vi "TCPcom.vi"(5 "string":string, 11 "error in":errorcluster, 13 "task":T1) -> (6 "data out":string, 15 "error out":errorcluster)   [LabVIEW 2020]
uses:
  task.ctl
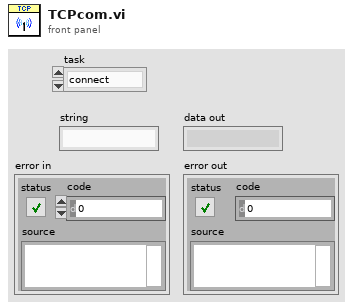
[diagram p1: front panel]
types:
  T1 = typedef "task.ctl" = enum16{"connect", "send", "send-recv", "receive", "disconnect"}
  T2 = enum16{"Standard", "Buffered", "CRLF", "Immediate"}
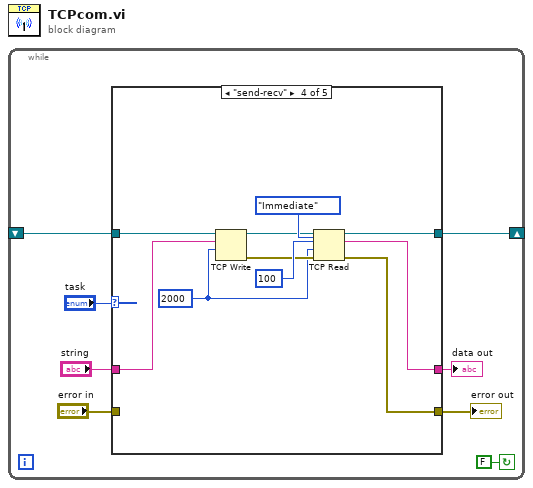
[diagram p0: block diagram]
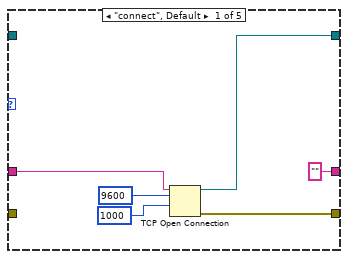
[diagram p2: hidden frame]
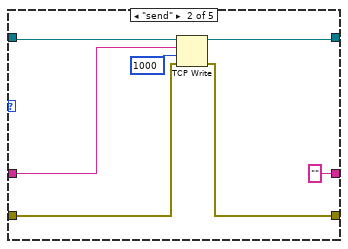
[diagram p3: hidden frame]
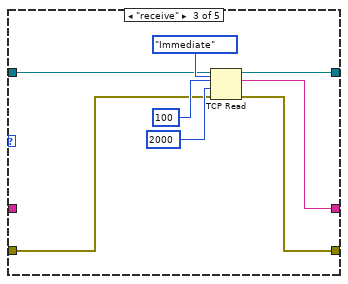
[diagram p4: hidden frame]
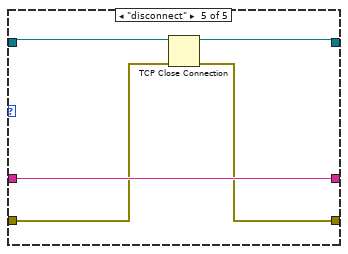
[diagram p5: hidden frame]
diagram:
  n1 = while {
    shift-right: [w7] -> _
    shift-left: _ -> [w6]
    stop <- FALSE continue-if-true
    n2 = case shown="\"send-recv\"" "task" {
      tunnel: [w10 w19 w27 w37 w42] -> w7
      tunnel: w6 -> [_ w20 w22 w34 w43]
      tunnel: "string" -> [w12 w16 _ w30 w44]
      tunnel: [w11 w17 w26 w36 w40] -> w3
      tunnel: ["" ("string") "" ("string") w25 w35 w44] -> w2
      tunnel: "error in" -> [_ w18 w23 _ w41]
      frame "connect", Default {
        n3 = TCP Open Connection(address=w12, remote port or service name=u16 9600, timeout ms (60000)=1000) -> (connection ID=w10:refnum<k5>, error out=w11:errorcluster)  [unwired: 2 in]
      }
      frame "send" {
        n4 = TCP Write(connection ID=w20, data in=w16, error in (no error)=w18, 9:1000 ("timeout ms (25000)")) -> (connection ID out=w19:refnum<k5>, error out=w17:errorcluster)  [unwired: 1 out]
      }
      frame "receive" {
        n5 = TCP Read(connection ID=w22, bytes to read=100, error in (no error)=w23, 7:T2."Immediate" ("mode (standard)"), 9:2000 ("timeout ms (25000)")) -> (connection ID out=w27:refnum<k5>, data out=w25:string, error out=w26:errorcluster)
      }
      frame "send-recv" {
        w31 = 2000 ("timeout ms (25000)")
        n6 = TCP Write(connection ID=w34, data in=w30, 9:w31) -> (connection ID out=w33:refnum<k5>, error out=w32:errorcluster)  [unwired: 1 in, 1 out]
        n7 = TCP Read(connection ID=w33, bytes to read=100, error in (no error)=w32, 7:T2."Immediate" ("mode (standard)"), 9:w31) -> (connection ID out=w37:refnum<k5>, data out=w35:string, error out=w36:errorcluster)
      }
      frame "disconnect" {
        n8 = TCP Close Connection(connection ID=w43, error in (no error)=w41) -> (connection ID out=w42:refnum<k5>, error out=w40:errorcluster)  [unwired: 1 in]
      }
    }
    "error out" <- w3
    "data out" <- w2
  }
